vi "USBData_measure_dummy.vi"(0 "USBData in":refnum<class "USBData.lvclass">, 5 "DAQ timeout":dbl, 7 "DAQ sample #":i64, 9 "MeasurementIndex":i64, 11 "error in (no error)":errorcluster) -> (1 "TimeMeasuremeent":timestamp, 3 "LastDataAcquired":dbl[](array[numeric]), 4 "USBData out":refnum<class "USBData.lvclass">, 6 "LabelLD":string, 8 "Labels":string[](array[string]), 10 "Status":T1(ring), 15 "error out":errorcluster)   [LabVIEW 2017, in "USBData.lvclass"]
uses:
  USBData.lvclass
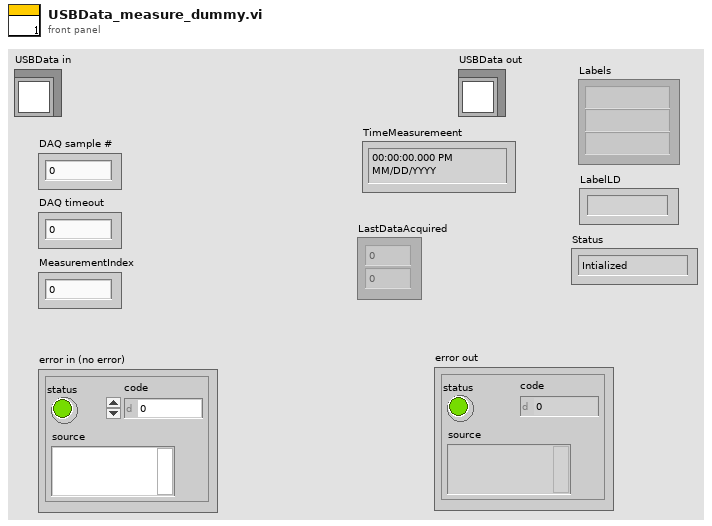
[diagram p1: front panel]
types:
  T1 = enum16{"Intialized", "Waiting", "Measuring", "Terminated"}
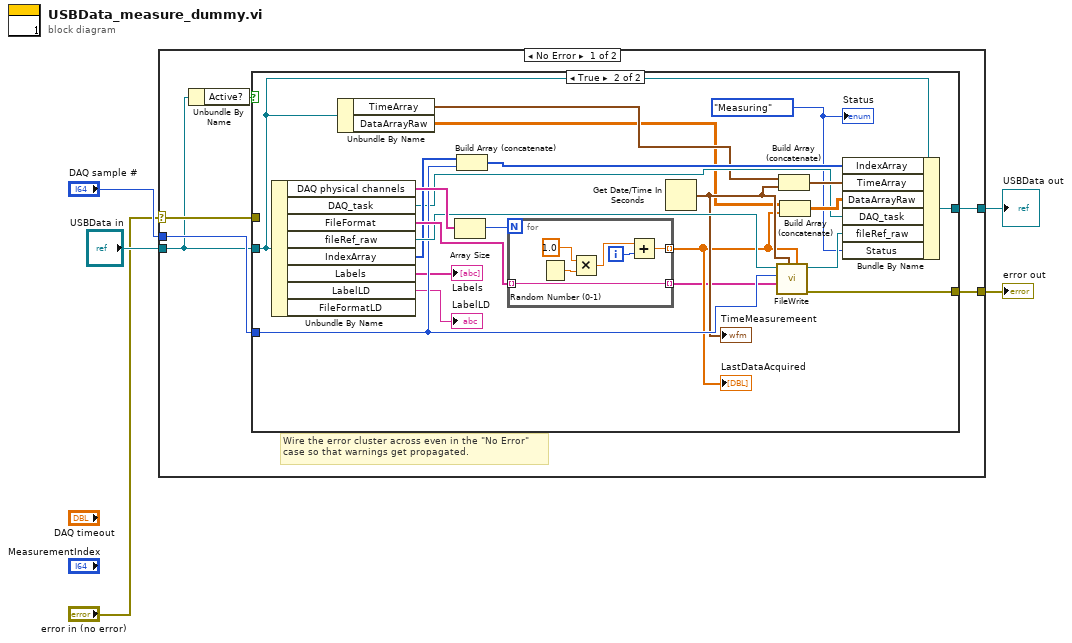
[diagram p0: block diagram]
diagram:
  n1 = case shown="No Error" "error in (no error)" {
    selector: "error in (no error)" -> [w7 w43]
    tunnel: [w10 w43] -> w5
    tunnel: "DAQ sample #" -> [w11 _]
    tunnel: [w8 w42] -> w3
    tunnel: "USBData in" -> [w6 w42]
    frame No Error {
      # "Wire the error cluster across even in the \"No Error\"\ncase so that warnings get propagated."
      n2 = Unbundle By Name(w6) -> ("Active?"=w9:bool)
      n3 = case shown="True" w9 {
        tunnel: [w12 w32] -> w10
        tunnel: w11 -> [_ w26]
        tunnel: [w13 w17] -> w8
        tunnel: w6 -> [w13 w16]
        tunnel: w7 -> [w12 _]
        frame False {
        }
        frame True {
          w20 = T1."Measuring" ("Status")
          n4 = Unbundle By Name(w16) -> ("DAQ physical channels"=w28:tag[], "DAQ_task"=w24:refnum<k21>, "FileFormat"=w33:string[], "fileRef_raw"=w27:refnum<file>, "IndexArray"=w25:i64[], "Labels"=→"Labels":string[], "LabelLD"=→"LabelLD":string)  [unwired: 1 out]
          n5 = Unbundle By Name(w16) -> ("TimeArray"=w15:timestamp[], "DataArrayRaw"=w14:dbl[][])
          n6 = Array Size(array=w28) -> (size(s)=w35:i32)
          n7 = Build Array (concatenate)(w25, w26) -> (w29:i64[])
          n8 = for {
            N: w35 -> [_]
            tunnel: w33 -> [w41] mode=indexing
            tunnel: [w41] -> w18 mode=indexing
            tunnel: [w36] -> w19 mode=indexing
            i -> [w37]
            n9 = Random Number (0-1)() -> (number: 0 to 1=w40:dbl)
            n10 = Multiply(x=1.0, y=w40) -> (x*y=w38:dbl)
            n11 = Add(x=w38, y=w37) -> (x+y=w36:dbl)
          }
          "LastDataAcquired" <- w19
          n12 = Get Date/Time In Seconds() -> (seconds since 1Jan1904=w21:timestamp)
          "TimeMeasuremeent" <- w21
          n13 = call "FileWrite.vi"("DataArray"=w19, "Time Stamp"=w21, "FileFormat"=w18, "Index"=w26, "refnum in"=w27) -> ("Error Out"=w32:errorcluster, "Byte Stream File Refnum"=w30:refnum<file>)  [unwired: 5 in]
          n14 = Build Array (concatenate)(w15, w21) -> (w34:timestamp[])
          n15 = Build Array (concatenate)(w14, w19) -> (w31:dbl[][])
          n16 = Bundle By Name(cluster=w16, "IndexArray"=w29, "TimeArray"=w34, "DataArrayRaw"=w31, "DAQ_task"=w24, "fileRef_raw"=w30, "Status"=w20) -> (w17:refnum<class "USBData.lvclass">)
          "Status" <- w20
        }
      }
    }
    frame Error {
    }
  }
  "error out" <- w5
  "USBData out" <- w3
